vi "Event Ctr, Falling Edge (SubVI).vi"(1 "Reset":bool, 2 "Trigger":bool) -> (0 "8-bit Count (0-63)":u8)   [LabVIEW 2016]
doc: "This VI supports a falling edge event counter. When the input trigger creates a falling edge, the value of 8-bit Count is incremented on the host VI."
panel:
  # "This VI supports a falling edge event counter.  When the input trigger creates a falling edge, the value of 8-bit Count is incremented on the host VI."
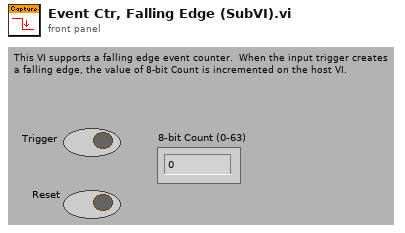
[diagram p1: front panel]
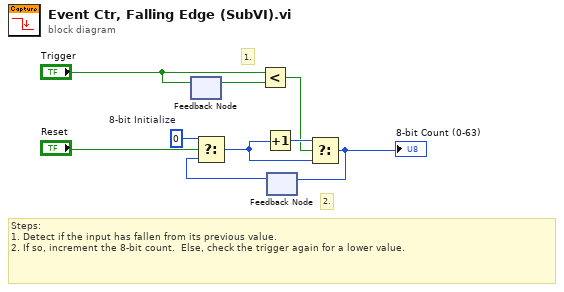
[diagram p0: block diagram]
diagram:
  w9 = u8 0  # 8-bit Initialize
  # "1."
  # "2."
  # "Steps:\n1. Detect if the input has fallen from its previous value.\n2. If so, increment the 8-bit count.  Else, check the trigger again for a lower value."
  n1 = feedback-in #1("Trigger") -> ()
  n2 = feedback #1() -> (w4:bool)  [unwired: 1 out]
  n3 = Less?(x="Trigger", y=w4) -> (x < y?=w6:bool)
  n4 = feedback #2() -> (w5:u8)  [unwired: 1 out]
  n5 = Select(t=w9, s="Reset", f=w5) -> (s? t:f=w8:u8)
  n6 = Increment(x=w8) -> (x+1=w7:u8)
  n7 = Select(t=w7, s=w6, f=w8) -> (s? t:f=w3:u8)
  "8-bit Count (0-63)" <- w3
  n8 = feedback-in #2(w3) -> ()
